vi "copy_method_change_input.vi"(8 "error in":errorcluster, 10 "name or relative path":string="config_data_cluster.ctl", 11 "new class reference in":refnum<vi>) -> (0 "error out":errorcluster, 1 "new vi path out":path, 3 "new class reference out":refnum<vi>, 5 "new class path out":path)   [LabVIEW 2010]
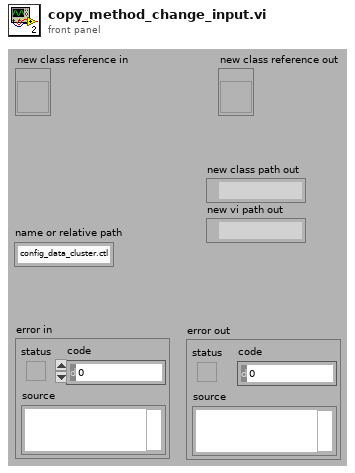
[diagram p1: front panel]
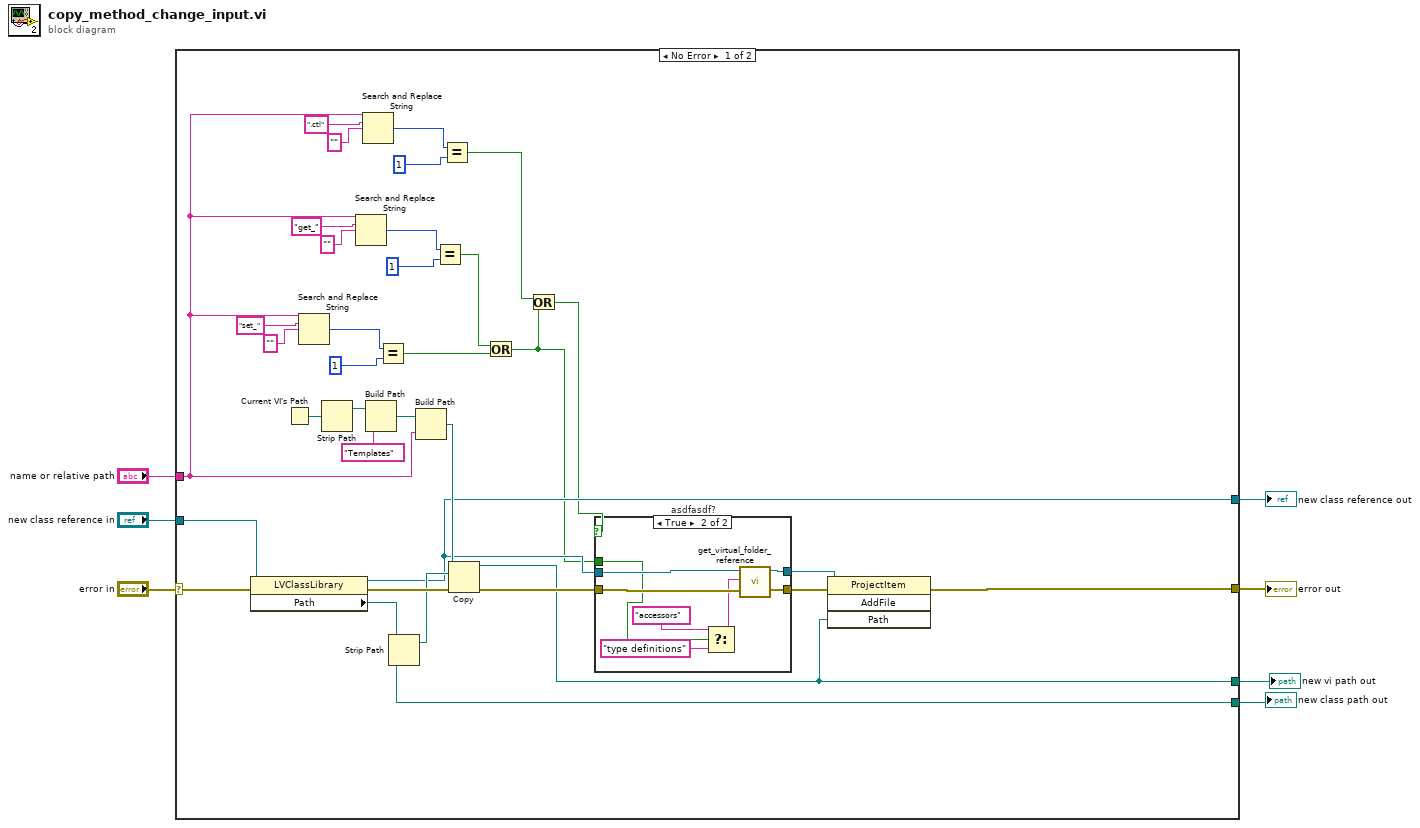
[diagram p0: block diagram]
diagram:
  n1 = case shown="No Error" "error in" {
    selector: "error in" -> [w33 w52]
    tunnel: [w8 w52] -> w7
    tunnel: [w16 w53] -> w3
    tunnel: "new class reference in" -> [w36 w53]
    tunnel: "name or relative path" -> [w17 _]
    tunnel: [w14 _] -> w2
    tunnel: [w15 _] -> w1
    frame No Error {
      n2 = property class="LVClassLibrary"(reference=w36, error in=w33) -> (reference out=w16:refnum<vi>, error out=w35:errorcluster, "Path"=w15:path)
      n3 = Current VI's Path() -> (path=w41:path)
      n4 = Search and Replace String(input string=w17, search string="set_", replace string="" ("replace string (\"\")")) -> (number of replacements=w25:i32)  [unwired: 5 in, 3 out]
      n5 = Strip Path(path=w41) -> (stripped path=w40:path)  [unwired: 1 out]
      n6 = Search and Replace String(input string=w17, search string="get_", replace string="" ("replace string (\"\")")) -> (number of replacements=w31:i32)  [unwired: 5 in, 3 out]
      n7 = Search and Replace String(input string=w17, search string=".ctl", replace string="" ("replace string (\"\")")) -> (number of replacements=w19:i32)  [unwired: 5 in, 3 out]
      n8 = Build Path(base path=w40, name or relative path="Templates") -> (appended path=w38:path)
      n9 = Equal?(x=w25, y=1) -> (x = y?=w23:bool)
      n10 = Strip Path(path=w15) -> (stripped path=w34:path)  [unwired: 1 out]
      n11 = Build Path(base path=w38, name or relative path=w17) -> (appended path=w37:path)
      n12 = Equal?(x=w31, y=1) -> (x = y?=w29:bool)
      n13 = Equal?(x=w19, y=1) -> (x = y?=w10:bool)
      n14 = Copy(8:w35, 10:w34, 11:w37) -> (0:w22:errorcluster, 3:w14:path)  [unwired: 2 in, 1 out]
      n15 = Or(x=w29, y=w23) -> (x .or. y?=w11:bool)
      n16 = Or(x=w10, y=w11) -> (x .or. y?=w9:bool)
      n17 = case "asdfasdf?" shown="True" w9 {
        tunnel: w11 -> [_ w47]
        tunnel: w22 -> [w42 w51]
        tunnel: w16 -> [w43 w50]
        tunnel: [w42 w49] -> w13
        tunnel: [w43 w48] -> w12
        frame False {
        }
        frame True {
          n18 = Select(t="accessors" ("name of virtual folder"), s=w47, f="type definitions") -> (s? t:f=w44:string)
          n19 = call "get_virtual_folder_reference.vi"("error in (no error)"=w51, "name of virtual folder"=w44, "new class reference in"=w50) -> ("error out"=w49:errorcluster, "virtual folder ref out"=w48:refnum<vi>)  [unwired: 6 in]
        }
      }
      n20 = invoke on="Invoke Node" class="ProjectItem" method="AddFile"(reference=w12, error in=w13, "Path"=w14) -> (error out=w8:errorcluster)  [unwired: 1 in, 3 out]
    }
    frame Error {
    }
  }
  "new class reference out" <- w3
  "error out" <- w7
  "new vi path out" <- w2
  "new class path out" <- w1
